vi "Check wavelength Validity.vi"(8 "error in (no error)":errorcluster, 11 "Wavelength string":string) -> (0 "Error Out (no error)":errorcluster)   [LabVIEW 2017]
panel:
  out "offset past scan":u32
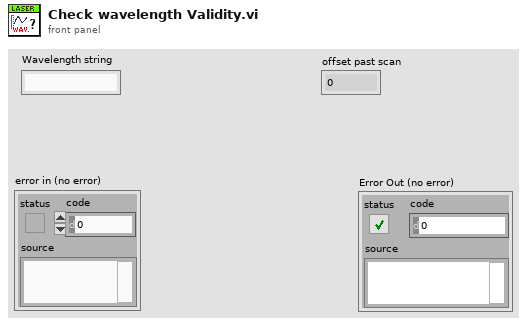
[diagram p1: front panel]
types:
  T1 = typedef "laser status data.ctl" = cluster{"Laser wavelength":i32, "Laser status":u8, "Motor Homing":bool, "Laser Shutter":bool, "Laser fault":u8, "Keyswitch":bool, "Change code":u8}
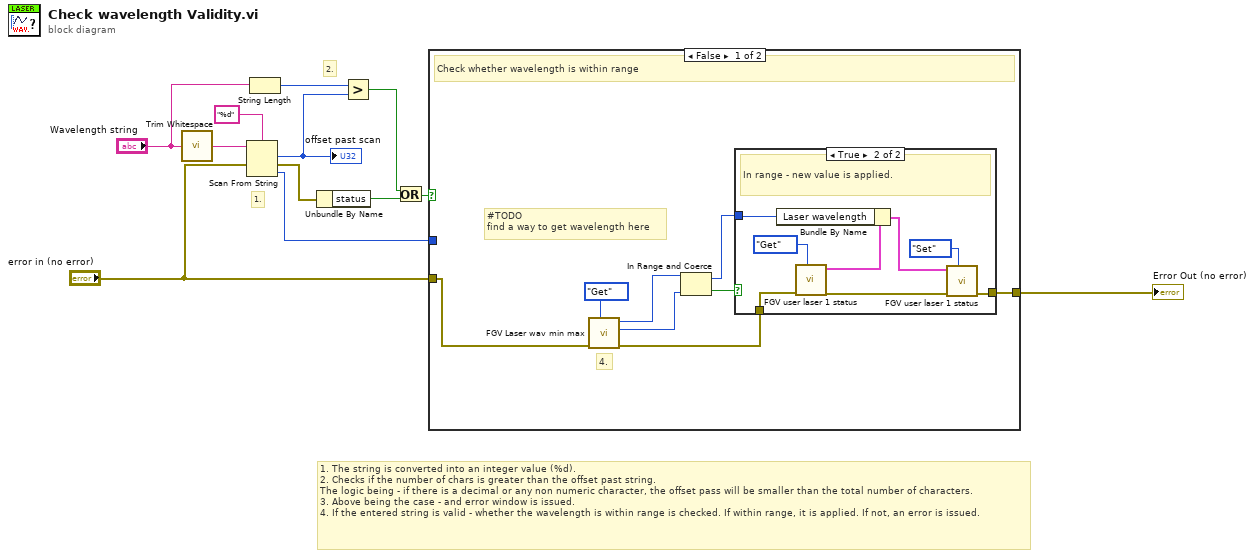
[diagram p0: block diagram]
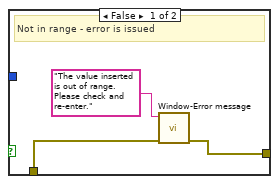
[diagram p2: hidden frame]
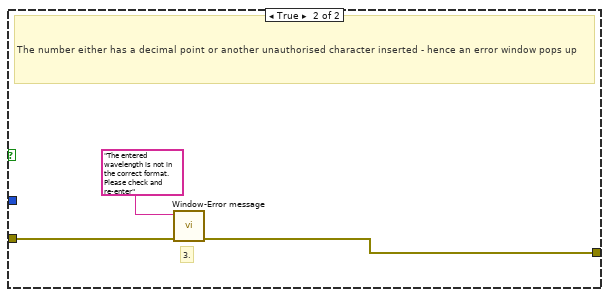
[diagram p3: hidden frame]
diagram:
  # "2."
  # "1. The string is converted into an integer value (%d).\n2. Checks if the number of chars is greater than the offset past string.\nThe logic being - if there is a decimal or any non numeric character, the offset pass will be smaller than the total number of characters.\n3. Above being the case - and error window is issued.\n4. If the entered string is valid - whether the wavelength is within range is checked. If within range, it is applied. If not, an error is issued."
  # "1."
  n1 = call <vilib>:"Trim Whitespace.vi"("string"="Wavelength string") -> ("trimmed string"=w12:string)  [unwired: 1 in]
  n2 = Scan From String(format string="%d", input string=w12, error in="error in (no error)") -> (offset past scan=w8:u32, error out=w7:errorcluster, output 1=w2:i32)  [unwired: 2 in, 1 out]
  "offset past scan" <- w8
  n3 = String Length(string="Wavelength string") -> (length=w9:i32)
  n4 = Unbundle By Name(w7) -> ("status"=w5:bool)
  n5 = Greater?(x=w9, y=w8) -> (0:w6:bool)
  n6 = Or(x=w6, y=w5) -> (x .or. y?=w4:bool)
  n7 = case shown="False" w4 {
    tunnel: "error in (no error)" -> [w20 w35]
    tunnel: [w13 w33] -> w1
    tunnel: w2 -> [_ _]
    frame False {
      # "#TODO \nfind a way to get wavelength here"
      # "4."
      # "Check whether wavelength is within range"
      n8 = call "FGV Laser wav min max.vi"("FGV Actions"=enum16{"Get", "Set"}."Get", "error in (no error)"=w20) -> ("error out"=w14:errorcluster, "Tmin Out"=w17:u16, "Tmax Out"=w18:u16)  [unwired: 7 in]
      n9 = In Range and Coerce(upper limit=w18, lower limit=w17) -> (x=w19:u16, coerced(x)=w15:u16, In Range?=w16:bool)
      n10 = case shown="True" w16 {
        tunnel: w15 -> [_ w29]
        tunnel: w14 -> [w24 w32]
        tunnel: [w22 w27] -> w13
        frame False {
          # "Not in range - error is issued"
          n11 = call "Window-Error message.vi"("error in (no error)"=w24, "Message"="The value inserted is out of range. Please check and re-enter.") -> ("Error Out (no error)"=w22:errorcluster)  [unwired: 9 in]
        }
        frame True {
          # "In range - new value is applied."
          n12 = call "FGV user laser 1 status.vi"("FGV Actions"=enum16{"Get", "Set"}."Get", "error in (no error)"=w32) -> ("error out"=w25:errorcluster, "Laser Status OUT"=w30:T1)  [unwired: 8 in]
          n13 = Bundle By Name(cluster=w30, "Laser wavelength"=w29) -> (w26:T1)
          n14 = call "FGV user laser 1 status.vi"("FGV Actions"=enum16{"Get", "Set"}."Set", "error in (no error)"=w25, "Laser status IN"=w26) -> ("error out"=w27:errorcluster)  [unwired: 7 in, 1 out]
        }
      }
    }
    frame True {
      # "3."
      # "The number either has a decimal point or another unauthorised character inserted - hence an error window pops up"
      n15 = call "Window-Error message.vi"("error in (no error)"=w35, "Message"="The entered wavelength is not in the correct format. Please check and re-enter") -> ("Error Out (no error)"=w33:errorcluster)  [unwired: 9 in]
    }
  }
  "Error Out (no error)" <- w1
